vi "U6 easy Stream Full with FFT.vi"() -> ()   [LabVIEW 2021]
uses:
  <vilib>/Analysis/NI_AALPro.lvlib
panel:
  out "RMS Voltage vs. Frequency":cluster{i32, dbl, dbl[][]}(graph)
  out "Voltage vs. Time":cluster{i32, dbl, dbl[][]}(graph)
  in  "Binary":bool
  in  "StreamSettlingFactor":i32
  in  "Resolution Index":u8
  in  "Range Constants":u8[](array[ring])=[0, 0] items=["LJ_rgBIP10V", "LJ_rgBIP1V", "LJ_rgBIPP1V", "LJ_rgBIPP01V"]
  out "Stream Parameters":T1 {"Device Backlog [%]" format="%.2f"}
  in  "PC buffer size (seconds)":dbl=10.0 format="%.2f"
  in  "Scan List (-)":u8[](array[numeric])=[199, 199]
  out "Data":dbl[][](array[numeric]) format="%.3f"
  in  "Scan List (+)":u8[](array[numeric])=[0, 1]
  out "# of iterations":i32
  in  "Scan Rate (Hz)":dbl=1024.0 format="%.3f"
  in  "stop":bool
  out "Error Message":string
  # "This example streams from the first found USB U6."
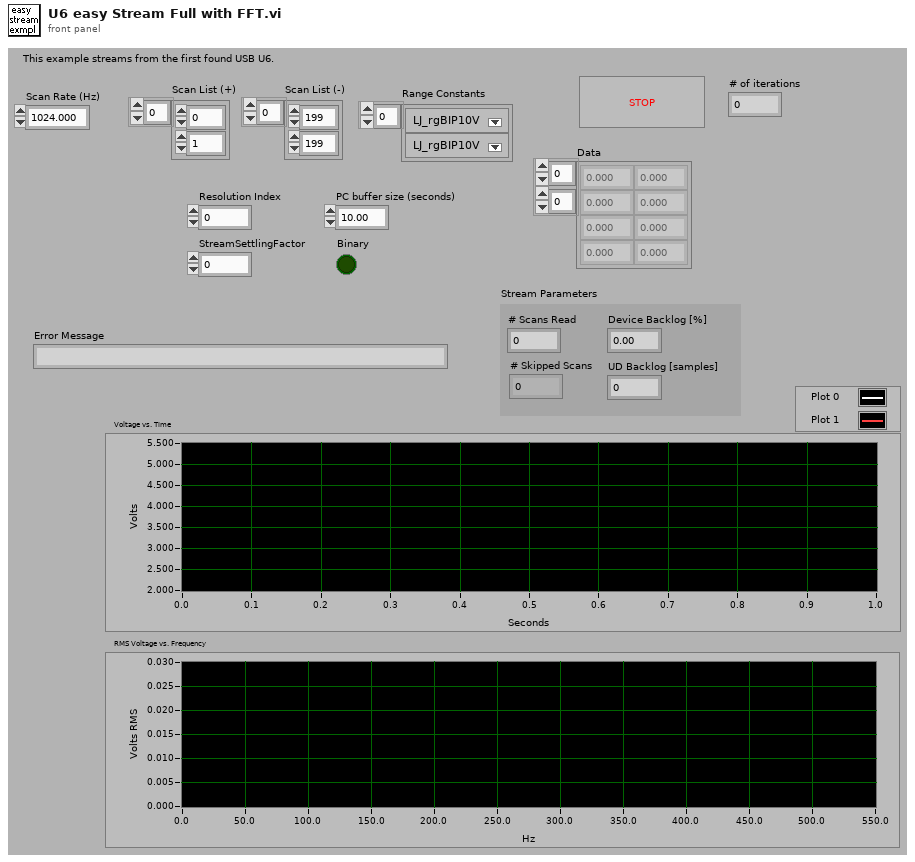
[diagram p1: front panel]
types:
  T1 = cluster{"# Scans Read":i32, "# Skipped Scans":i32, "Device Backlog [%]":dbl, "UD Backlog [samples]":i32}
  T2 = cluster{"PC buffer size (seconds)":dbl, "Resolution Index":u8, "StreamSettlingFactor":i32, "Binary":bool}
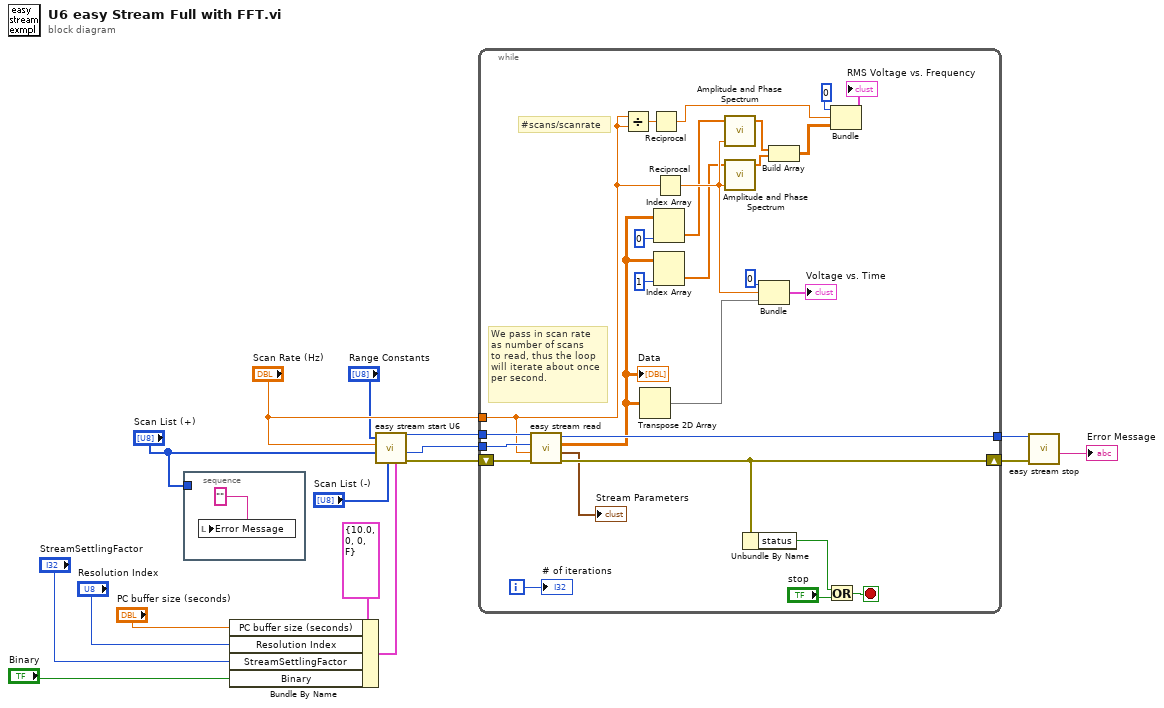
[diagram p0: block diagram]
diagram:
  n1 = stacked-sequence {
    tunnel: "Scan List (+)" -> [_]
    frame #0 {
      n2 = local write "Error Message"("" ("Error Message")) -> ()
    }
  }
  n3 = Bundle By Name(cluster=T2 {"PC buffer size (seconds)"=10.0, "Resolution Index"=0, "StreamSettlingFactor"=0, "Binary"=FALSE} ("Advanced"), "PC buffer size (seconds)"="PC buffer size (seconds)", "Resolution Index"="Resolution Index", "StreamSettlingFactor"="StreamSettlingFactor", "Binary"="Binary") -> (w5:T2)
  n4 = call "easy stream start U6.vi"("Advanced"=w5, "Scan List (-)"="Scan List (-)", "Scan List (+)"="Scan List (+)", "Scan Rate (Hz)"="Scan Rate (Hz)", "Range Constants"="Range Constants") -> ("error out"=w16:errorcluster, "# Channels"=w15:i32, "Handle Out"=w14:i32)  [unwired: 3 in, 1 out]
  n5 = while {
    tunnel: "Scan Rate (Hz)" -> [w18]
    tunnel: [w37] -> w12
    tunnel: w14 -> [w38]
    tunnel: w15 -> [w39]
    shift-left: w16 -> [w40]
    shift-right: [w36] -> w13
    i -> [w41]
    stop <- w42 stop-if-true
    # "#scans/scanrate"
    # "We pass in scan rate\nas number of scans\nto read, thus the loop\nwill iterate about once\nper second."
    n6 = call "easy stream read.vi"("error in"=w40, "Scans To Read"=w18, "# Channels In Stream"=w39, "Handle In"=w38) -> ("error out"=w36:errorcluster, "Stream Parameters"=→"Stream Parameters":T1, "Data"=w19:dbl[][], "Handle Out"=w37:i32)  [unwired: 4 in]
    "Data" <- w19
    n7 = Divide(x=w18, y=w18) -> (x/y=w26:dbl)
    n8 = Transpose 2D Array(2D array=w19) -> (transposed array=w21:dbl[][])
    n9 = Reciprocal(x=w26) -> (1/x=w29:dbl)
    n10 = Index Array(array=w19, index (col)=0 ("Index")) -> (element=w30:dbl[])  [unwired: 1 in]
    n11 = Index Array(array=w19, index (col)=1 ("Index")) -> (element=w25:dbl[])  [unwired: 1 in]
    n12 = Reciprocal(x=w18) -> (1/x=w34:dbl)
    n13 = call <vilib>:"Amplitude and Phase Spectrum.vi"("dt"=w34, "Signal (V)"=w30) -> ("Amp Spectrum Mag (Vrms)"=w31:dbl[])  [unwired: 1 in, 2 out]
    n14 = call <vilib>:"Amplitude and Phase Spectrum.vi"("dt"=w34, "Signal (V)"=w25) -> ("Amp Spectrum Mag (Vrms)"=w27:dbl[])  [unwired: 1 in, 2 out]
    n15 = Unbundle By Name(w36) -> ("status"=w43:bool)
    n16 = Bundle(0, w34, w21) -> (→"Voltage vs. Time":cluster{i32, dbl, dbl[][]})  [unwired: 1 in]
    n17 = Build Array(w31, w27) -> (w32:dbl[][])
    n18 = Or(x=w43, y="stop") -> (x .or. y?=w42:bool)
    n19 = Bundle(0, w29, w32) -> (→"RMS Voltage vs. Frequency":cluster{i32, dbl, dbl[][]})  [unwired: 1 in]
    "# of iterations" <- w41
  }
  n20 = call "easy stream stop.vi"("error in"=w13, "Handle In"=w12) -> ("Error Message"=→"Error Message":string)  [unwired: 7 in, 2 out]
